vi "Appearance Read.vi"(4 "error in (no error)":errorcluster, 6 "Container State":T3, 7 "Display State In":T2) -> (0 "error out":errorcluster, 2 "Value":T1, 3 "Display State Out":T2)   [LabVIEW 2015]
uses:
  <vilib>/_xctls/Container State.ctl
  State.ctl
  <vilib>/_xctls/XControlSupport.lvlib
  Stimulus Channel (V3).xctl
panel:
  # "Replace the Value Indicator below with an Indicator of desired type.\nDo not remove this Indicator or the others from the connector pane. \nDo not change the connector pane pattern.\nThe Value Indicator should always be the second terminal from top on the output side in the connector pane."
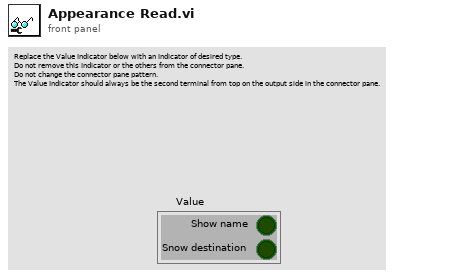
[diagram p1: front panel]
types:
  T1 = cluster{"Show name":bool, "Snow destination":bool}
  T2 = typedef "Stimulus Channel (V3).xctl/State.ctl" = cluster{"Show advanced":bool, "Show rove":bool, "Show name":bool, "Show dest":bool, "Lock dest":bool, "Dests":string[], "max level":dbl, "LMax Event":refnum<user-event>}
  T3 = typedef "XControlSupport.lvlib/Container State.ctl" = cluster{"Indicator?":bool, "Run Mode?":bool, " Refnum":refnum<vi>}
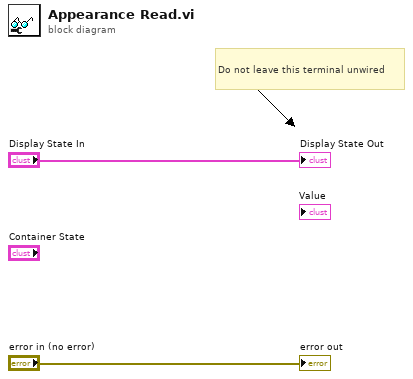
[diagram p0: block diagram]
diagram:
  # "Do not leave this terminal unwired"
  "error out" <- "error in (no error)"
  "Display State Out" <- "Display State In"
